vi "Init.vi"(8 "error in (no error)":errorcluster, 9 "Search Offset (0)":i32, 10 "Source Name":string, 11 "Scene Name":string) -> (0 "error out":errorcluster, 3 "GetSceneItemID out":refnum<class "GetSceneItemID.lvclass">)   [LabVIEW 2022 SP3, in "obs-websocket-lv.lvlib" / "GetSceneItemID.lvclass"]
uses:
  GetSceneItemID.lvclass
  GetSceneItemID.lvclass/GetSceneItemID.ctl
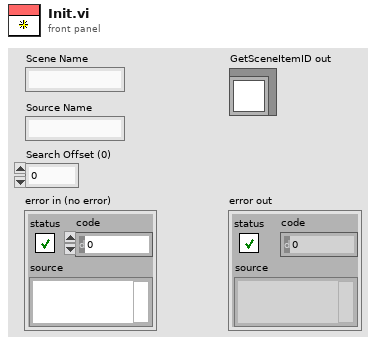
[diagram p1: front panel]
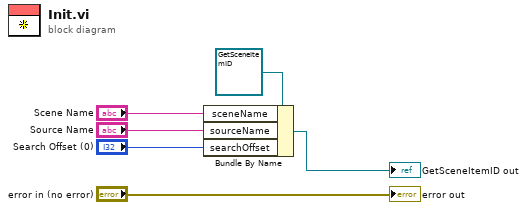
[diagram p0: block diagram]
diagram:
  n1 = Bundle By Name(cluster=refnum<class "GetSceneItemID.lvclass"> refnum ("GetSceneItemID in"), "sceneName"="Scene Name", "sourceName"="Source Name", "searchOffset"="Search Offset (0)") -> (→"GetSceneItemID out":refnum<class "GetSceneItemID.lvclass">)
  "error out" <- "error in (no error)"
